vi "Parameter Analyzer Config.vi"() -> (0 "HP4155C Configuration":T1={"Parameter Analyzer VISA Session"="COM1", "Sweeping Time Parameters"={"Integration Time"=0, "Short Integration Time (s)"=1.0, "Long Integration Time (s)"=0.0, "Wait Time Parameter"=1.0}, "Acquisition Mode"=enum."Sweeping Mode", "Status Polling Time (ms)"=1000, "Comment"="Test VI", "SMU 1 - Sweeping"={"Start / Offset"=0.0, "Stop / Ratio"=1.0, "Step \n(linear only)"=0.01, "Compliance"=0.1, "Power \nCompliance"=0.0, "Mode"=0, "Function"=0, "Sweep Mode"=FALSE}, "SMU 2 - Sweeping"={"Start / Offset"=0.0, "Stop / Ratio"=1.0, "Step \n(linear only)"=0.01, "Compliance"=0.1, "Power \nCompliance"=0.0, "Mode"=0, "Function"=0, "Sweep Mode"=FALSE}, "SMU 3 - Sweeping"={"Start / Offset"=0.0, "Stop / Ratio"=1.0, "Step \n(linear only)"=0.01, "Compliance"=0.1, "Power \nCompliance"=0.0, "Mode"=0, "Function"=0, "Sweep Mode"=FALSE}, "SMU 4 - Sweeping"={"Start / Offset"=0.0, "Stop / Ratio"=1.0, "Step \n(linear only)"=0.01, "Compliance"=0.1, "Power \nCompliance"=0.0, "Mode"=0, "Function"=0, "Sweep Mode"=FALSE}, "Sweep Spacing"=0, "Range"=0, "SMU1 - Sampling"={"Source"=10.0, "Compliance"=1e-05, "Mode"=0, "Function"=FALSE}, "SMU2 - Sampling"={"Source"=10.0, "Compliance"=1e-05, "Mode"=0, "Function"=FALSE}, "SMU3 - Sampling"={"Source"=10.0, "Compliance"=1e-05, "Mode"=0, "Function"=FALSE}, "SMU4 - Sampling"={"Source"=10.0, "Compliance"=1e-05, "Mode"=0, "Function"=FALSE}, "Sampling Time Parameters"={"Initial Interval (s)"=0.1, "Number of Samples"=60, "Total Sampling Time (s)"=10.0, "Hold Time (s)"=0.0, "Sampling Mode"=0, "Sampling Time"=0}, "Stop Condition"={"Enable Delay (s)"=0.0, "Name"="", "Threshold"=0.0, "num. of events"=1, "Event"=0, "Stop Condition Enable"=FALSE}} {"Stop Condition"."Event" items=["Value > Threshold", "Value < Threshold", "| Value | > | Threshold |", "| Value | < | Threshold |"]; "Stop Condition"."Threshold" format="%^.2e"; "Stop Condition"."Enable Delay (s)" format="%.1f"; "Sampling Time Parameters"."Sampling Time" items=["Auto (linear only)", "No Limit", "Set Limit"]; "Sampling Time Parameters"."Sampling Mode" items=["Linear", "Log10", "Log25", "Log50", "Thinned Out"]; "Sampling Time Parameters"."Hold Time (s)" format="%.4f"; "Sampling Time Parameters"."Total Sampling Time (s)" format="%.1f"; "Sampling Time Parameters"."Initial Interval (s)" format="%^.3e"; "SMU 4 - Sweeping"."Function" items=["Disabled", "Var 1", "Var 2", "Var 1'", "Constant"]; "SMU 4 - Sweeping"."Mode" items=["V", "I", "V pulse", "I  pulse", "Common"]; "SMU 4 - Sweeping"."Power \nCompliance" format="%^.2e"; "SMU 4 - Sweeping"."Compliance" format="%^.2e"; "SMU 4 - Sweeping"."Step \n(linear only)" format="%^.4e"; "SMU 4 - Sweeping"."Stop / Ratio" format="%^.4e"; "SMU 4 - Sweeping"."Start / Offset" format="%^.4e"; "SMU 3 - Sweeping"."Function" items=["Disabled", "Var 1", "Var 2", "Var 1'", "Constant"]; "SMU 3 - Sweeping"."Mode" items=["V", "I", "V pulse", "I  pulse", "Common"]; "SMU 3 - Sweeping"."Power \nCompliance" format="%^.2e"; "SMU 3 - Sweeping"."Compliance" format="%^.2e"; "SMU 3 - Sweeping"."Step \n(linear only)" format="%^.4e"; "SMU 3 - Sweeping"."Stop / Ratio" format="%^.4e"; "SMU 3 - Sweeping"."Start / Offset" format="%^.4e"; "SMU 2 - Sweeping"."Function" items=["Disabled", "Var 1", "Var 2", "Var 1'", "Constant"]; "SMU 2 - Sweeping"."Mode" items=["V", "I", "V pulse", "I  pulse", "Common"]; "SMU 2 - Sweeping"."Power \nCompliance" format="%^.2e"; "SMU 2 - Sweeping"."Compliance" format="%^.2e"; "SMU 2 - Sweeping"."Step \n(linear only)" format="%^.4e"; "SMU 2 - Sweeping"."Stop / Ratio" format="%^.4e"; "SMU 2 - Sweeping"."Start / Offset" format="%^.4e"; "SMU 1 - Sweeping"."Function" items=["Disabled", "Var 1", "Var 2", "Var 1'", "Constant"]; "SMU 1 - Sweeping"."Mode" items=["V", "I", "V pulse", "I  pulse", "Common"]; "SMU 1 - Sweeping"."Power \nCompliance" format="%^.2e"; "SMU 1 - Sweeping"."Compliance" format="%^.2e"; "SMU 1 - Sweeping"."Step \n(linear only)" format="%^.4e"; "SMU 1 - Sweeping"."Stop / Ratio" format="%^.4e"; "SMU 1 - Sweeping"."Start / Offset" format="%^.4e"; "Sweeping Time Parameters"."Long Integration Time (s)" scale=0.02..2.0; "Sweeping Time Parameters"."Short Integration Time (s)" scale=8e-05..0.00192; "Sweeping Time Parameters"."Integration Time" items=["Short", "Long"]; "Sweeping Time Parameters"."Wait Time Parameter" format="%.1f"; "SMU4 - Sampling"."Mode" items=["V", "I", "Common"]; "SMU4 - Sampling"."Compliance" format="%^.2e"; "SMU4 - Sampling"."Source" format="%^.3e"; "SMU3 - Sampling"."Mode" items=["V", "I", "Common"]; "SMU3 - Sampling"."Compliance" format="%^.2e"; "SMU3 - Sampling"."Source" format="%^.3e"; "SMU2 - Sampling"."Mode" items=["V", "I", "Common"]; "SMU2 - Sampling"."Compliance" format="%^.2e"; "SMU2 - Sampling"."Source" format="%^.3e"; "SMU1 - Sampling"."Mode" items=["V", "I", "Common"]; "SMU1 - Sampling"."Compliance" format="%^.2e"; "SMU1 - Sampling"."Source" format="%^.3e"; "Range" items=["auto", "fixed", "limited"]; "Sweep Spacing" items=["linear", "log 10", "log 25", "log 50"]})   [LabVIEW 2014]
uses:
  Parameter Analyzer Config.ctl
  Parameter Analyzer Integration Parameters.ctl
  Parameter Analyzer SMU Sweeping.ctl
  Parameter Analyzer Sweep Spacing.ctl
  Parameter Analyzer SMU Range.ctl
  Parameter Analyzer SMU Sampling.ctl
  Parameter Analyzer Sampling Parameters.ctl
  Parameter Analyzer Stop Sampling Conditions.ctl
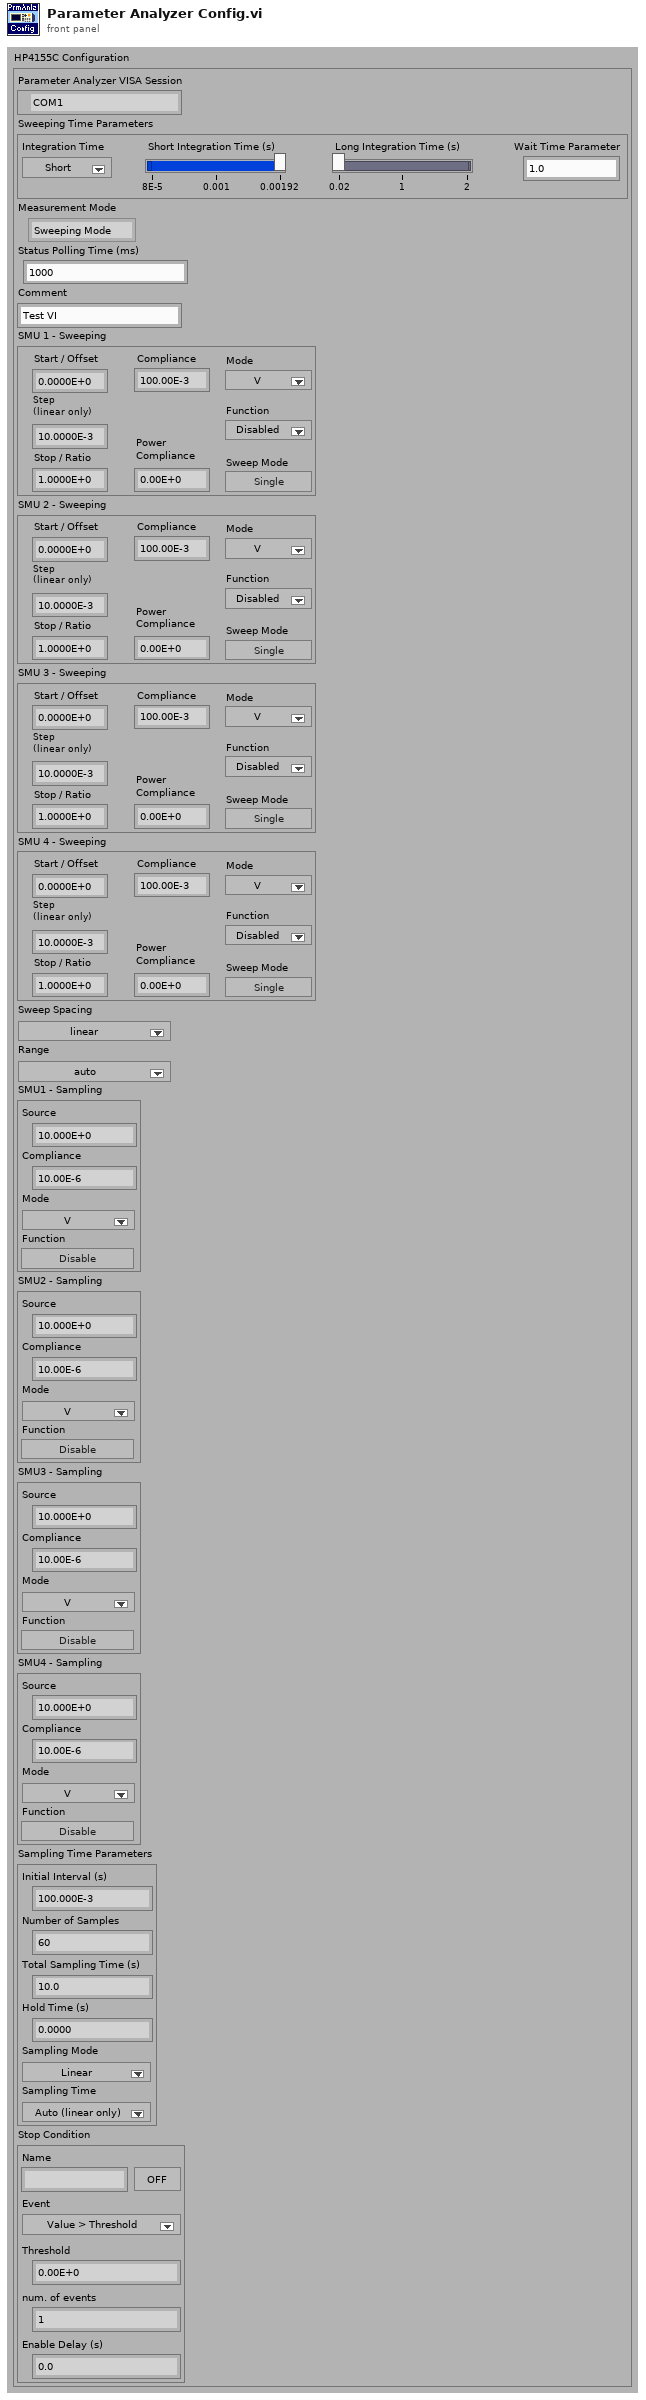
[diagram p1: front panel]
types:
  T1 = typedef "Parameter Analyzer Config.ctl" = cluster{"Parameter Analyzer VISA Session":refnum<visa-resource-name>, "Sweeping Time Parameters":T2, "Acquisition Mode":enum32{"Sweeping Mode", "Sampling Mode"}, "Status Polling Time (ms)":u32, "Comment":string, "SMU 1 - Sweeping":T3, "SMU 2 - Sweeping":T3, "SMU 3 - Sweeping":T3, "SMU 4 - Sweeping":T3, "Sweep Spacing":T4, "Range":T5, "SMU1 - Sampling":T6, "SMU2 - Sampling":T6, "SMU3 - Sampling":T6, "SMU4 - Sampling":T6, "Sampling Time Parameters":T7, "Stop Condition":T8}
  T2 = typedef "Parameter Analyzer Integration Parameters.ctl" = cluster{"Integration Time":u32, "Short Integration Time (s)":dbl, "Long Integration Time (s)":dbl, "Wait Time Parameter":dbl}
  T3 = typedef "Parameter Analyzer SMU Sweeping.ctl" = cluster{"Start / Offset":dbl, "Stop / Ratio":dbl, "Step \n(linear only)":dbl, "Compliance":dbl, "Power \nCompliance":dbl, "Mode":u32, "Function":i32, "Sweep Mode":bool}
  T4 = typedef "Parameter Analyzer Sweep Spacing.ctl" = u16
  T5 = typedef "Parameter Analyzer SMU Range.ctl" = u16
  T6 = typedef "Parameter Analyzer SMU Sampling.ctl" = cluster{"Source":dbl, "Compliance":dbl, "Mode":u32, "Function":bool}
  T7 = typedef "Parameter Analyzer Sampling Parameters.ctl" = cluster{"Initial Interval (s)":dbl, "Number of Samples":i32, "Total Sampling Time (s)":dbl, "Hold Time (s)":dbl, "Sampling Mode":i32, "Sampling Time":i32}
  T8 = typedef "Parameter Analyzer Stop Sampling Conditions.ctl" = cluster{"Enable Delay (s)":dbl, "Name":string, "Threshold":dbl, "num. of events":i32, "Event":i32, "Stop Condition Enable":bool}
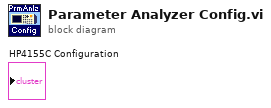
[diagram p0: block diagram]
diagram:
